vi "Read_Timestamp.vi"(8 "error in (no error)":errorcluster, 10 "Lower Timestamp Limit":i64, 11 "Upper Timestamp Limit":i64=3) -> (0 "error out":errorcluster, 1 "Experiment Settings Array":T3[](array[typedef]), 2 "Dust Signal Array":T2[](array[typedef]), 3 "Pelletron Array":T4[](array[typedef]), 5 "Dust Event Array":T1[](array[typedef]))   [LabVIEW 2011]
uses:
  <vilib>/addons/database/NI_Database_API.lvlib
  <vilib>/addons/database/Auxilliary.llb/DB Tools Cursor Type.ctl
  Pelletron.ctl
  <vilib>/addons/database/_DB Variant To Data/Database Variant To Data.xnode
  <vilib>/addons/database/Connection.llb/Conn Execute.vi
  <vilib>/addons/database/Recordset.llb/Rec Fetch Recordset Data (R).vi
  <vilib>/addons/database/Recordset.llb/Rec Destroy - Connection.vi
  Public API/ExperimentSetting.ctl
  Public API/Post_Dust_Event.ctl
  Public API/Post_Signal.ctl
panel:
  out "Dust Event size(s)":i32
  out "Dust Signal size(s)":i32
  out "Experiment Settings size(s)":i32
  out "Experiment Settings SQL Query Sintax":string
  out "Dust Signal SQL Query Sintax":string
  out "Dust Event SQL Query Sintax":string
  out "Pelletron Array size(s)":i32
  out "Pelletron SQL Query Sintax":string
  # "Dust Event"
  # "Signal"
  # "Experiment Settings"
  # "Pelletron"
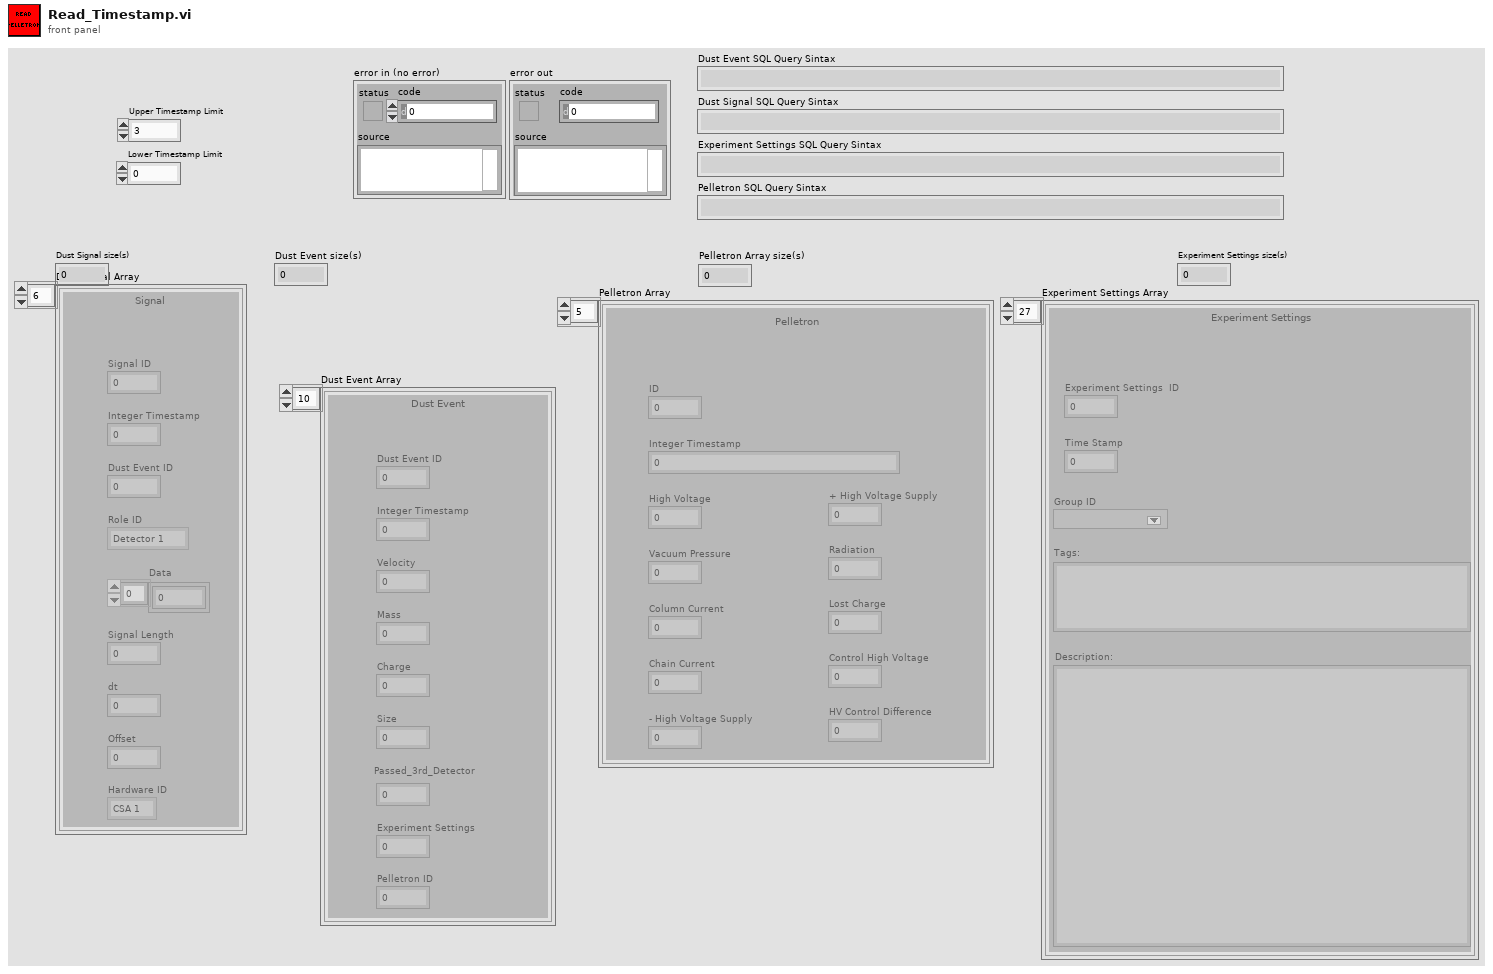
[diagram p1: front panel]
types:
  T1 = typedef "Post_Dust_Event.ctl" = cluster{"Dust Event ID":i64, "Integer Timestamp":i64, "Velocity":sgl, "Mass":sgl, "Charge":sgl, "Size":sgl, "Passed_3rd_Detector":i8, "Experiment Settings":dbl, "Pelletron ID":i32}
  T2 = typedef "Post_Signal.ctl" = cluster{"Signal ID":i64, "Integer Timestamp":i64, "Dust Event ID":i64, "Role ID":enum16{"Detector 1", "Reserved", "Detector 2", "Final Detector"}, "Data":sgl[], "Signal Length":i32, "dt":i64, "Offset":dbl, "Hardware ID":enum16{"CSA 1", "CSA 2", "CSA 3", "CSA 4", "CSA 5", "CSA 6"}}
  T3 = typedef "ExperimentSetting.ctl" = cluster{"Experiment Settings  ID":i64, "Time Stamp":i64, "Group ID":i32, "Tags:":string, "Description:":string}
  T4 = typedef "Pelletron.ctl" = cluster{"ID":i32, "Integer Timestamp":u64, "High Voltage":sgl, "+ High Voltage Supply":sgl, "- High Voltage Supply":sgl, "HV Control Difference":sgl, "Vacuum Pressure":sgl, "Radiation":sgl, "Column Current":sgl, "Lost Charge":sgl, "Chain Current":sgl, "Control High Voltage":sgl}
  T5 = typedef "NI_Database_API.lvlib/DB Tools Cursor Type.ctl" = enum16{"forward-only", "keyset", "dynamic", "static"}
  T6 = typedef "NI_Database_API.lvlib/Conn ObjectReference.ctl" = refnum<k1>
  T7 = typedef "NI_Database_API.lvlib/Rec ObjectReference.ctl" = refnum<k1>
  T8 = enum16{"Detector 1", "Reserved", "Detector 2", "Final Detector"}
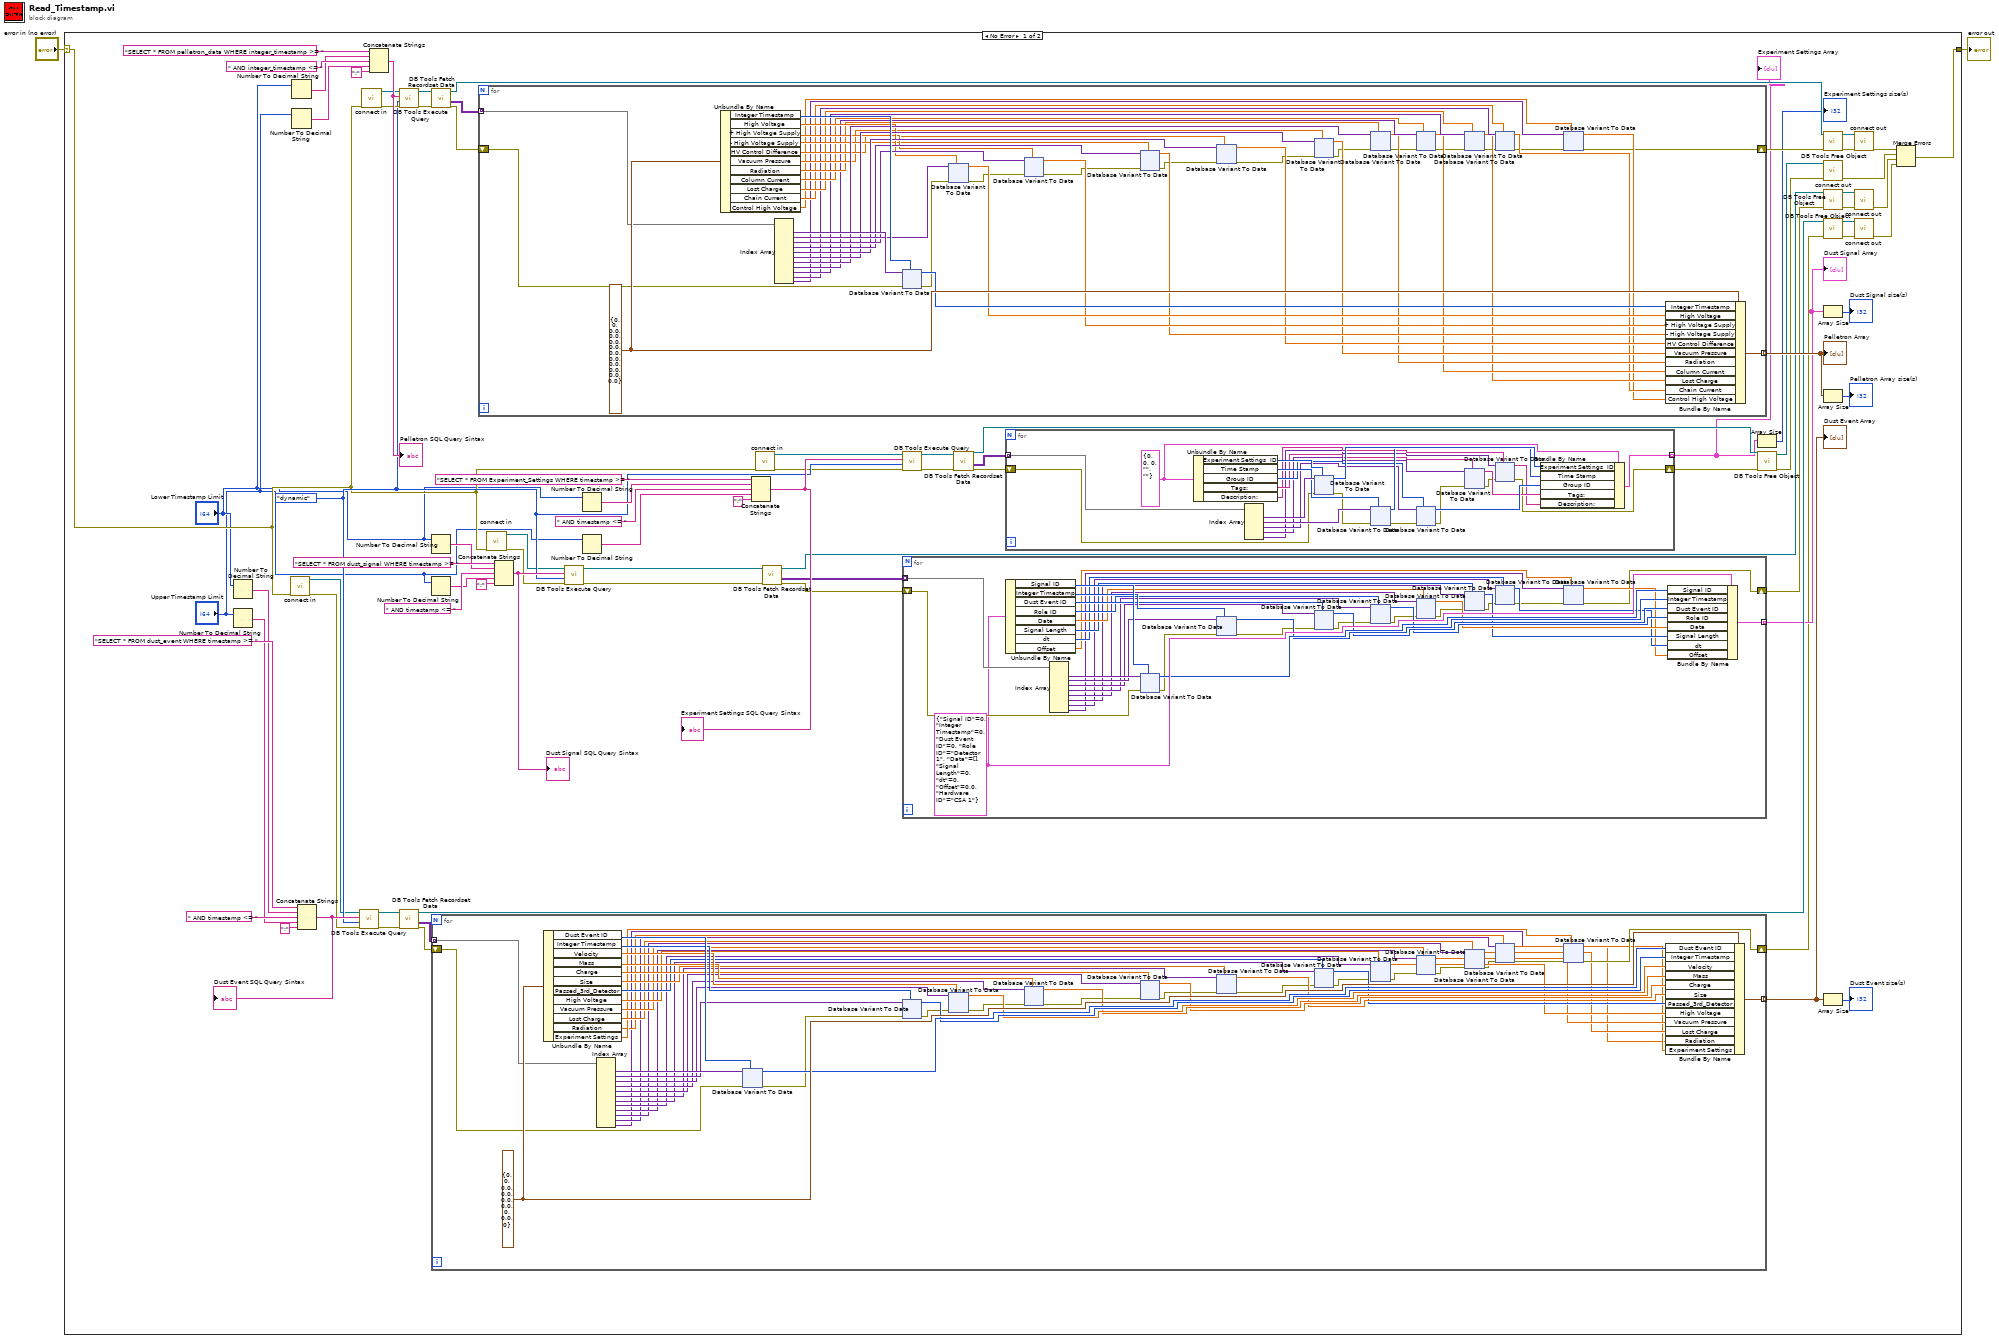
[diagram p0: block diagram]
diagram:
  n1 = case shown="No Error" "error in (no error)" {
    selector: "error in (no error)" -> [w30 w1399]
    tunnel: [w23 w1399] -> w1
    frame No Error {
      w42 = DB_Tools_Cursor_Type."dynamic" ("cursor type")
      n2 = Number To Decimal String(number="Lower Timestamp Limit") -> (decimal integer string=w67:string)  [unwired: 1 in]
      n3 = Number To Decimal String(number="Upper Timestamp Limit") -> (decimal integer string=w66:string)  [unwired: 1 in]
      n4 = call "connect in.vi"("error in (no error)"=w30) -> ("error out"=w29:errorcluster, "Database Connection"=w28:T6)  [unwired: 6 in, 1 out]
      n5 = Number To Decimal String(number="Lower Timestamp Limit") -> (decimal integer string=w76:string)  [unwired: 1 in]
      n6 = Number To Decimal String(number="Upper Timestamp Limit") -> (decimal integer string=w74:string)  [unwired: 1 in]
      n7 = Concatenate Strings("SELECT * FROM dust_event WHERE timestamp >= " ("string"), w67, " AND timestamp <= " ("string"), w66, ";" ("string")) -> (w45:string)
      "Dust Event SQL Query Sintax" <- w45
      n8 = call-poly <vilib>:"DB Tools Execute Query.vi"("error in (no error)"=w29, "cursor type"=w42, "SQL query"=w45, "connection reference"=w28) -> ("error out"=w54:errorcluster, "recordset reference"=w55:T7)  [unwired: 4 in]
      n9 = call "connect in.vi"("error in (no error)"=w30) -> ("error out"=w46:errorcluster, "Database Connection"=w48:T6)  [unwired: 6 in, 1 out]
      n10 = Concatenate Strings("SELECT * FROM pelletron_data WHERE integer_timestamp >= " ("string"), w76, " AND integer_timestamp <= " ("string"), w74, ";" ("string")) -> (w80:string)
      "Pelletron SQL Query Sintax" <- w80
      n11 = call-poly <vilib>:"DB Tools Execute Query.vi"("error in (no error)"=w46, "cursor type"=w42, "SQL query"=w80, "connection reference"=w48) -> ("error out"=w77:errorcluster, "recordset reference"=w78:T7)  [unwired: 4 in]
      n12 = call-poly <vilib>:"DB Tools Fetch Recordset Data.vi"("error in (no error)"=w54, "recordset reference"=w55) -> ("error out"=w9:errorcluster, "recordset data"=w7:variant[][], "recordset reference out"=w39:T7)  [unwired: 3 in]
      n13 = call-poly <vilib>:"DB Tools Fetch Recordset Data.vi"("error in (no error)"=w77, "recordset reference"=w78) -> ("error out"=w47:errorcluster, "recordset data"=w75:variant[][], "recordset reference out"=w49:T7)  [unwired: 3 in]
      n14 = Number To Decimal String(number="Lower Timestamp Limit") -> (decimal integer string=w62:string)  [unwired: 1 in]
      n15 = Number To Decimal String(number="Upper Timestamp Limit") -> (decimal integer string=w61:string)  [unwired: 1 in]
      n16 = for {
        shift-right: [w132] -> w8
        shift-left: w9 -> [w133]
        tunnel: w7 -> [w134] mode=indexing
        tunnel: [w117] -> w5 mode=indexing
        w135 = T1 {"Dust Event ID"=0, "Integer Timestamp"=0, "Velocity"=0.0, "Mass"=0.0, "Charge"=0.0, "Size"=0.0, "Passed_3rd_Detector"=0, "Experiment Settings"=0.0, "Pelletron ID"=0} ("Cluster")
        n17 = Unbundle By Name(w135) -> ("Dust Event ID"=w131:i64, "Integer Timestamp"=w128:i64, "Velocity"=w125:sgl, "Mass"=w122:sgl, "Charge"=w119:sgl, "Size"=w115:sgl, "Passed_3rd_Detector"=w112:i8, "High Voltage"=w109:sgl, "Vacuum Pressure"=w107:sgl, "Lost Charge"=w103:sgl, "Radiation"=w99:sgl, "Experiment Settings"=w100:dbl)
        n18 = Index Array(array=w134) -> (element #1=w95:variant, element #2=w94:variant, element #3=w93:variant, element #4=w92:variant, element #5=w91:variant, element #6=w90:variant, element #7=w89:variant, element #8=w88:variant, element #9=w87:variant, element #10=w86:variant, element #11=w85:variant, element #12=w84:variant)  [unwired: 12 in]
        n19 = xnode "Database Variant To Data"("database variant"=w95, "error in"=w133, "type"=w131) -> ("data"=w130:i64, "error out"=w129:errorcluster)
        n20 = xnode "Database Variant To Data"("database variant"=w94, "error in"=w129, "type"=w128) -> ("data"=w127:i64, "error out"=w126:errorcluster)
        n21 = xnode "Database Variant To Data"("database variant"=w93, "error in"=w126, "type"=w125) -> ("data"=w124:sgl, "error out"=w123:errorcluster)
        n22 = xnode "Database Variant To Data"("database variant"=w92, "error in"=w123, "type"=w122) -> ("data"=w121:sgl, "error out"=w120:errorcluster)
        n23 = xnode "Database Variant To Data"("database variant"=w91, "error in"=w120, "type"=w119) -> ("data"=w118:sgl, "error out"=w116:errorcluster)
        n24 = xnode "Database Variant To Data"("database variant"=w90, "error in"=w116, "type"=w115) -> ("data"=w114:sgl, "error out"=w113:errorcluster)
        n25 = xnode "Database Variant To Data"("database variant"=w89, "error in"=w113, "type"=w112) -> ("data"=w111:i8, "error out"=w110:errorcluster)
        n26 = xnode "Database Variant To Data"("database variant"=w88, "error in"=w110, "type"=w109) -> ("data"=w108:sgl, "error out"=w105:errorcluster)
        n27 = xnode "Database Variant To Data"("database variant"=w87, "error in"=w105, "type"=w107) -> ("data"=w106:sgl, "error out"=w104:errorcluster)
        n28 = xnode "Database Variant To Data"("database variant"=w86, "error in"=w104, "type"=w103) -> ("data"=w102:sgl, "error out"=w96:errorcluster)
        n29 = xnode "Database Variant To Data"("database variant"=w85, "error in"=w96, "type"=w99) -> ("data"=w98:sgl, "error out"=w97:errorcluster)
        n30 = xnode "Database Variant To Data"("database variant"=w84, "error in"=w97, "type"=w100) -> ("data"=w101:dbl, "error out"=w132:errorcluster)
        n31 = Bundle By Name(cluster=w135, "Dust Event ID"=w130, "Integer Timestamp"=w127, "Velocity"=w124, "Mass"=w121, "Charge"=w118, "Size"=w114, "Passed_3rd_Detector"=w111, "High Voltage"=w108, "Vacuum Pressure"=w106, "Lost Charge"=w102, "Radiation"=w98, "Experiment Settings"=w101) -> (w117:T1)
      }
      "Dust Event Array" <- w5
      n32 = for {
        tunnel: w75 -> [w1045] mode=indexing
        tunnel: [w1001] -> w72 mode=indexing
        shift-right: [w999] -> w73
        shift-left: w47 -> [w1000]
        w1046 = T4 {"ID"=0, "Integer Timestamp"=0, "High Voltage"=0.0, "+ High Voltage Supply"=0.0, "- High Voltage Supply"=0.0, "HV Control Difference"=0.0, "Vacuum Pressure"=0.0, "Radiation"=0.0, "Column Current"=0.0, "Lost Charge"=0.0, "Chain Current"=0.0, "Control High Voltage"=0.0} ("Cluster")
        n33 = Unbundle By Name(w1046) -> ("Integer Timestamp"=w1044:u64, "High Voltage"=w1034:sgl, "+ High Voltage Supply"=w1033:sgl, "- High Voltage Supply"=w1032:sgl, "HV Control Difference"=w1031:sgl, "Vacuum Pressure"=w1030:sgl, "Radiation"=w1029:sgl, "Column Current"=w1028:sgl, "Lost Charge"=w1027:sgl, "Chain Current"=w1026:sgl, "Control High Voltage"=w1025:sgl)
        n34 = Index Array(array=w1045) -> (element #1=w1042:variant, element #2=w1041:variant, element #3=w1040:variant, element #4=w1039:variant, element #5=w1038:variant, element #6=w1037:variant, element #7=w1036:variant, element #8=w1024:variant, element #9=w1023:variant, element #10=w1022:variant, element #11=w1021:variant)  [unwired: 11 in]
        n35 = xnode "Database Variant To Data"("database variant"=w1042, "error in"=w1000, "type"=w1044) -> ("data"=w1043:u64, "error out"=w1011:errorcluster)
        n36 = xnode "Database Variant To Data"("database variant"=w1041, "error in"=w1011, "type"=w1034) -> ("data"=w1035:sgl, "error out"=w1010:errorcluster)
        n37 = xnode "Database Variant To Data"("database variant"=w1040, "error in"=w1010, "type"=w1033) -> ("data"=w1020:sgl, "error out"=w1009:errorcluster)
        n38 = xnode "Database Variant To Data"("database variant"=w1039, "error in"=w1009, "type"=w1032) -> ("data"=w1019:sgl, "error out"=w1008:errorcluster)
        n39 = xnode "Database Variant To Data"("database variant"=w1038, "error in"=w1008, "type"=w1031) -> ("data"=w1018:sgl, "error out"=w1007:errorcluster)
        n40 = xnode "Database Variant To Data"("database variant"=w1037, "error in"=w1007, "type"=w1030) -> ("data"=w1017:sgl, "error out"=w1006:errorcluster)
        n41 = xnode "Database Variant To Data"("database variant"=w1036, "error in"=w1006, "type"=w1029) -> ("data"=w1016:sgl, "error out"=w1005:errorcluster)
        n42 = xnode "Database Variant To Data"("database variant"=w1024, "error in"=w1005, "type"=w1028) -> ("data"=w1015:sgl, "error out"=w1004:errorcluster)
        n43 = xnode "Database Variant To Data"("database variant"=w1023, "error in"=w1004, "type"=w1027) -> ("data"=w1014:sgl, "error out"=w1003:errorcluster)
        n44 = xnode "Database Variant To Data"("database variant"=w1022, "error in"=w1003, "type"=w1026) -> ("data"=w1013:sgl, "error out"=w1002:errorcluster)
        n45 = xnode "Database Variant To Data"("database variant"=w1021, "error in"=w1002, "type"=w1025) -> ("data"=w1012:sgl, "error out"=w999:errorcluster)
        n46 = Bundle By Name(cluster=w1046, "Integer Timestamp"=w1043, "High Voltage"=w1035, "+ High Voltage Supply"=w1020, "- High Voltage Supply"=w1019, "HV Control Difference"=w1018, "Vacuum Pressure"=w1017, "Radiation"=w1016, "Column Current"=w1015, "Lost Charge"=w1014, "Chain Current"=w1013, "Control High Voltage"=w1012) -> (w1001:T4)
      }
      "Pelletron Array" <- w72
      n47 = call "connect in.vi"("error in (no error)"=w30) -> ("error out"=w32:errorcluster, "Database Connection"=w31:T6)  [unwired: 6 in, 1 out]
      n48 = Concatenate Strings("SELECT * FROM dust_signal WHERE timestamp >= " ("string"), w62, " AND timestamp <= " ("string"), w61, ";" ("string")) -> (w44:string)
      "Dust Signal SQL Query Sintax" <- w44
      n49 = call-poly <vilib>:"DB Tools Execute Query.vi"("error in (no error)"=w32, "cursor type"=w42, "SQL query"=w44, "connection reference"=w31) -> ("error out"=w52:errorcluster, "recordset reference"=w53:T7)  [unwired: 4 in]
      n50 = Number To Decimal String(number="Lower Timestamp Limit") -> (decimal integer string=w57:string)  [unwired: 1 in]
      n51 = Number To Decimal String(number="Upper Timestamp Limit") -> (decimal integer string=w56:string)  [unwired: 1 in]
      n52 = Concatenate Strings("SELECT * FROM Experiment_Settings WHERE timestamp >= " ("string"), w57, " AND timestamp <= " ("string"), w56, ";" ("string")) -> (w43:string)
      "Experiment Settings SQL Query Sintax" <- w43
      n53 = call "connect in.vi"("error in (no error)"=w30) -> ("error out"=w34:errorcluster, "Database Connection"=w33:T6)  [unwired: 6 in, 1 out]
      n54 = call-poly <vilib>:"DB Tools Fetch Recordset Data.vi"("error in (no error)"=w52, "recordset reference"=w53) -> ("error out"=w13:errorcluster, "recordset data"=w14:variant[][], "recordset reference out"=w40:T7)  [unwired: 3 in]
      n55 = call-poly <vilib>:"DB Tools Execute Query.vi"("error in (no error)"=w34, "cursor type"=w42, "SQL query"=w43, "connection reference"=w33) -> ("error out"=w50:errorcluster, "recordset reference"=w51:T7)  [unwired: 4 in]
      n56 = for {
        tunnel: w14 -> [w555] mode=indexing
        shift-right: [w521] -> w12
        shift-left: w13 -> [w552]
        tunnel: [w520] -> w10 mode=indexing
        w551 = T2 {"Signal ID"=0, "Integer Timestamp"=0, "Dust Event ID"=0, "Role ID"=enum."Detector 1", "Data"=[], "Signal Length"=0, "dt"=0, "Offset"=0.0, "Hardware ID"=enum."CSA 1"} ("Post_Signal 2")
        n57 = Unbundle By Name(w551) -> ("Signal ID"=w554:i64, "Integer Timestamp"=w549:i64, "Dust Event ID"=w545:i64, "Role ID"=w541:T8, "Data"=w536:sgl[], "Signal Length"=w532:i32, "dt"=w528:i64, "Offset"=w523:dbl)
        n58 = Index Array(array=w555) -> (element #1=w553:variant, element #2=w548:variant, element #3=w544:variant, element #4=w540:variant, element #5=w537:variant, element #6=w533:variant, element #7=w529:variant, element #8=w524:variant)  [unwired: 8 in]
        n59 = xnode "Database Variant To Data"("database variant"=w553, "error in"=w552, "type"=w554) -> ("data"=w550:i64, "error out"=w547:errorcluster)
        n60 = xnode "Database Variant To Data"("database variant"=w548, "error in"=w547, "type"=w549) -> ("data"=w546:i64, "error out"=w543:errorcluster)
        n61 = xnode "Database Variant To Data"("database variant"=w544, "error in"=w543, "type"=w545) -> ("data"=w542:i64, "error out"=w539:errorcluster)
        n62 = xnode "Database Variant To Data"("database variant"=w540, "error in"=w539, "type"=w541) -> ("data"=w538:T8, "error out"=w534:errorcluster)
        n63 = xnode "Database Variant To Data"("database variant"=w537, "error in"=w534, "type"=w536) -> ("data"=w535:sgl[], "error out"=w530:errorcluster)
        n64 = xnode "Database Variant To Data"("database variant"=w533, "error in"=w530, "type"=w532) -> ("data"=w531:i32, "error out"=w526:errorcluster)
        n65 = xnode "Database Variant To Data"("database variant"=w529, "error in"=w526, "type"=w528) -> ("data"=w527:i64, "error out"=w525:errorcluster)
        n66 = xnode "Database Variant To Data"("database variant"=w524, "error in"=w525, "type"=w523) -> ("data"=w522:dbl, "error out"=w521:errorcluster)
        n67 = Bundle By Name(cluster=w551, "Signal ID"=w550, "Integer Timestamp"=w546, "Dust Event ID"=w542, "Role ID"=w538, "Data"=w535, "Signal Length"=w531, "dt"=w527, "Offset"=w522) -> (w520:T2)
      }
      "Dust Signal Array" <- w10
      n68 = call-poly <vilib>:"DB Tools Fetch Recordset Data.vi"("error in (no error)"=w50, "recordset reference"=w51) -> ("error out"=w18:errorcluster, "recordset data"=w19:variant[][], "recordset reference out"=w41:T7)  [unwired: 3 in]
      n69 = for {
        tunnel: w19 -> [w838] mode=indexing
        shift-right: [w816] -> w17
        shift-left: w18 -> [w821]
        tunnel: [w815] -> w15 mode=indexing
        w837 = T3 {"Experiment Settings  ID"=0, "Time Stamp"=0, "Group ID"=0, "Tags:"="", "Description:"=""} ("Experiment Settings")
        n70 = Unbundle By Name(w837) -> ("Experiment Settings  ID"=w835:i64, "Time Stamp"=w832:i64, "Group ID"=w829:i32, "Tags:"=w826:string, "Description:"=w824:string)
        n71 = Index Array(array=w838) -> (element #1=w836:variant, element #2=w833:variant, element #3=w830:variant, element #4=w827:variant, element #5=w823:variant)  [unwired: 5 in]
        n72 = xnode "Database Variant To Data"("database variant"=w836, "error in"=w821, "type"=w835) -> ("data"=w834:i64, "error out"=w820:errorcluster)
        n73 = xnode "Database Variant To Data"("database variant"=w833, "error in"=w820, "type"=w832) -> ("data"=w831:i64, "error out"=w819:errorcluster)
        n74 = xnode "Database Variant To Data"("database variant"=w830, "error in"=w819, "type"=w829) -> ("data"=w828:i32, "error out"=w818:errorcluster)
        n75 = xnode "Database Variant To Data"("database variant"=w827, "error in"=w818, "type"=w826) -> ("data"=w825:string, "error out"=w817:errorcluster)
        n76 = xnode "Database Variant To Data"("database variant"=w823, "error in"=w817, "type"=w824) -> ("data"=w822:string, "error out"=w816:errorcluster)
        n77 = Bundle By Name(cluster=w837, "Experiment Settings  ID"=w834, "Time Stamp"=w831, "Group ID"=w828, "Tags:"=w825, "Description:"=w822) -> (w815:T3)
      }
      "Experiment Settings Array" <- w15
      n78 = Array Size(array=w15) -> (size(s)=→"Experiment Settings size(s)":i32)
      n79 = call-poly <vilib>:"DB Tools Free Object.vi"("error in (no error)"=w17, "recordset reference"=w41) -> ("error out"=w25:errorcluster, "connection reference"=w37:T6)  [unwired: 8 in]
      n80 = call-poly <vilib>:"DB Tools Free Object.vi"("error in (no error)"=w73, "recordset reference"=w49) -> ("error out"=w79:errorcluster, "connection reference"=w38:T6)  [unwired: 8 in]
      n81 = call "connect out.vi"("error in (no error)"=w25, "connection reference"=w37) -> ("error out"=w22:errorcluster)  [unwired: 9 in]
      n82 = call-poly <vilib>:"DB Tools Free Object.vi"("error in (no error)"=w12, "recordset reference"=w40) -> ("error out"=w26:errorcluster, "connection reference"=w35:T6)  [unwired: 8 in]
      n83 = call-poly <vilib>:"DB Tools Free Object.vi"("error in (no error)"=w8, "recordset reference"=w39) -> ("error out"=w27:errorcluster, "connection reference"=w36:T6)  [unwired: 8 in]
      n84 = Array Size(array=w10) -> (size(s)=→"Dust Signal size(s)":i32)
      n85 = Array Size(array=w72) -> (size(s)=→"Pelletron Array size(s)":i32)
      n86 = Array Size(array=w5) -> (size(s)=→"Dust Event size(s)":i32)
      n87 = call "connect out.vi"("error in (no error)"=w79, "connection reference"=w38) -> ("error out"=w24:errorcluster)  [unwired: 9 in]
      n88 = call "connect out.vi"("error in (no error)"=w26, "connection reference"=w35) -> ("error out"=w21:errorcluster)  [unwired: 9 in]
      n89 = call "connect out.vi"("error in (no error)"=w27, "connection reference"=w36) -> ("error out"=w20:errorcluster)  [unwired: 9 in]
      n90 = Merge Errors(w24, w22, w21, w20) -> (w23:errorcluster)
    }
    frame Error {
    }
  }
  "error out" <- w1
